vi "set_FPGA_reference.vi"(8 "error in (no error)":errorcluster, 10 "FPGA VI Reference":T1) -> (0 "error out":errorcluster)   [LabVIEW 2010, in "FPGAWrapperRK110512Fiber_Spiral.lvclass"]
uses:
  FPGAWrapperRK110512Fiber_Spiral.lvclass
  FPGA_VI_Reference.ctl
  class_data.vi
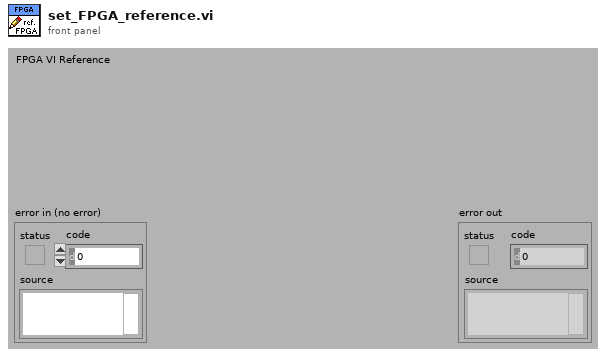
[diagram p1: front panel]
types:
  T1 = typedef "FPGAWrapperRK110512Fiber_Spiral.lvclass/FPGA_VI_Reference.ctl" = refnum<k20>
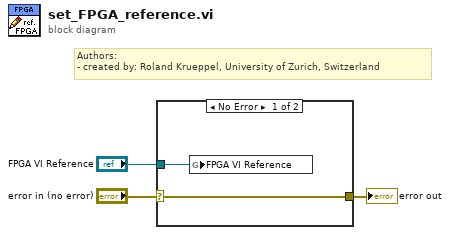
[diagram p0: block diagram]
diagram:
  # "Authors: \n- created by: Roland Krueppel, University of Zurich, Switzerland"
  n1 = case shown="No Error" "error in (no error)" {
    selector: "error in (no error)" -> [w5 w6]
    tunnel: [w5 w6] -> w2
    tunnel: "FPGA VI Reference" -> [w4 _]
    frame No Error {
      n2 = global write "class_data.vi" "FPGA VI Reference"(w4) -> ()
    }
    frame Error {
    }
  }
  "error out" <- w2
